vi "RemoveStatus Display Messages.vi"(10 "Numeric":i32, 11 "Status Display Array":string[](array[string])) -> (3 "array w/ subset deleted":string[](array[string]))   [LabVIEW 2011]
uses:
  <userlib>/_OpenG.lib/array/array.llb/Delete Elements from 1D Array (String)__ogtk.vi
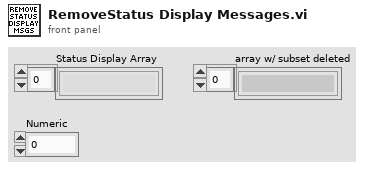
[diagram p1: front panel]
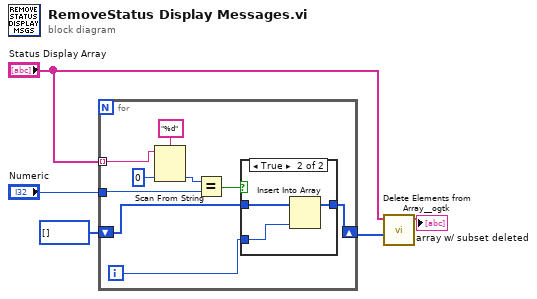
[diagram p0: block diagram]
diagram:
  n1 = for {
    tunnel: "Status Display Array" -> [w12] mode=indexing
    tunnel: "Numeric" -> [w10]
    shift-right: [w6] -> w3
    shift-left: i32[] [] -> [w8]
    i -> [w7]
    n2 = Scan From String(format string="%d", input string=w12, default 1=0) -> (output 1=w11:i32)  [unwired: 2 in, 3 out]
    n3 = Equal?(x=w11, y=w10) -> (x = y?=w9:bool)
    n4 = case shown="True" w9 {
      tunnel: w8 -> [w15 w18]
      tunnel: w7 -> [_ w17]
      tunnel: [w15 w16] -> w6
      frame False {
      }
      frame True {
        n5 = Insert Into Array(array=w18, new element=w17) -> (w16:i32[])  [unwired: 1 in]
      }
    }
  }
  n6 = call-poly <userlib>:"Delete Elements from Array__ogtk.vi"("indices"=w3, "array"="Status Display Array") -> ("array w/ subset deleted"=→"array w/ subset deleted":string[])  [unwired: 8 in, 1 out]
